vi "online image analysis and update.vi"(11 "Image in":T1) -> ()   [LabVIEW 2011, in "MoveDataFile.lvclass"]
uses:
  MoveDataFile.lvclass
  <vilib>/vision/Image Controls.llb/IMAQ Image.ctl
  shared/CompressAndUpdate(Poly)/CompressAndUpdate(Numeric).vi
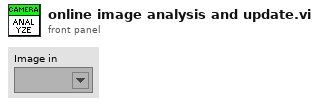
[diagram p1: front panel]
types:
  T1 = typedef "IMAQ Image.ctl" = refnum<image>
  T2 = typedef "Image analysys result.ctl" = cluster{"CentroidX":sgl, "CentroidY":sgl, "MeanCounts":sgl, "FWHMx":sgl, "FWHMy":sgl, "MaxCounts":sgl}
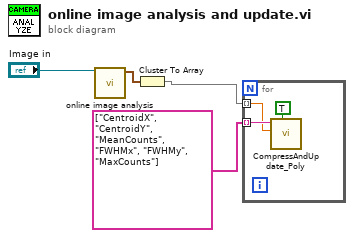
[diagram p0: block diagram]
diagram:
  n1 = call "online image analysis.vi"("Refnum in"="Image in") -> ("Image Analysis Result"=w2:T2)  [unwired: 10 in]
  n2 = Cluster To Array(cluster=w2) -> (array=w4:sgl[])
  n3 = for {
    tunnel: string[] ["CentroidX", "CentroidY", "MeanCounts", "FWHMx", "FWHMy", "MaxCounts"] -> [w6] mode=indexing
    tunnel: w4 -> [w5] mode=indexing
    n4 = call-poly "CompressAndUpdate_Poly.vi"("force CVT update (false)"=TRUE, "Numeric"=w5, "command or variable name"=w6) -> ()  [unwired: 8 in, 1 out]
  }
